vi "Test_Build.vi"() -> ()   [LabVIEW 2019]
uses:
  <vilib>/Platform/fileVersionInfo.llb/FileVersionInformation.ctl
panel:
  out "Application Path out":path
  out "FileVersionInfo Out":T1
  out "File Version Info":string
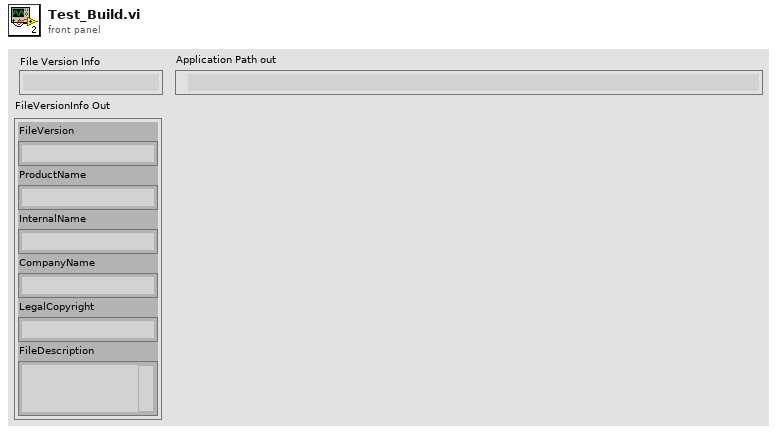
[diagram p1: front panel]
types:
  T1 = typedef "FileVersionInformation.ctl" = cluster{"FileVersion":string, "ProductName":string, "InternalName":string, "CompanyName":string, "LegalCopyright":string, "FileDescription":string}
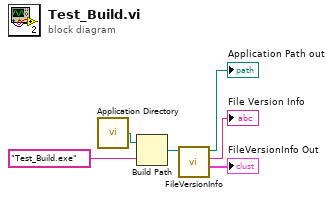
[diagram p0: block diagram]
diagram:
  n1 = call <vilib>:"Application Directory.vi"() -> ("Application Directory"=w3:path)
  n2 = Build Path(base path=w3, name or relative path="Test_Build.exe") -> (appended path=w2:path)
  n3 = call <vilib>:"FileVersionInfo.vi"("Application Path in"=w2) -> ("FileVersionInfo Out"=→"FileVersionInfo Out":T1, "File Version Info"=→"File Version Info":string, "Application Path out"=→"Application Path out":path)  [unwired: 7 in, 1 out]
